vi "Clear.vi"(8 "error in (no error)":errorcluster, 11 "Image in":refnum<class "Image.lvclass">) -> (0 "error out":errorcluster, 3 "Image out":refnum<class "Image.lvclass">)   [LabVIEW 2020, in "RPI.SenseHat.Display.lvlib" / "Image.lvclass"]
doc: "Fills the image with black color."
uses:
  Image.lvclass
  Color/Color.lvclass
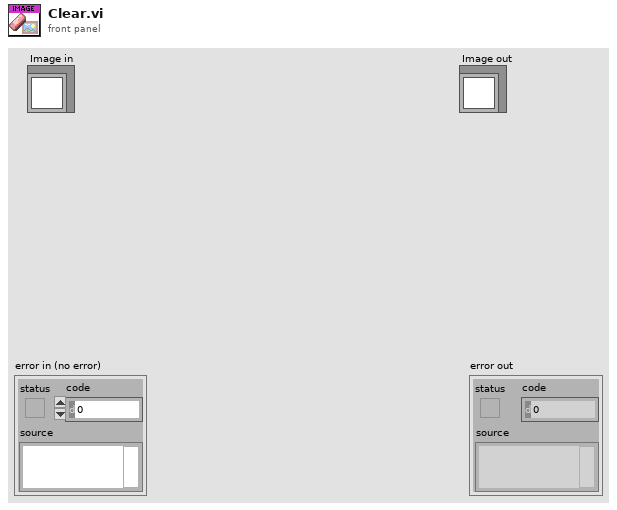
[diagram p1: front panel]
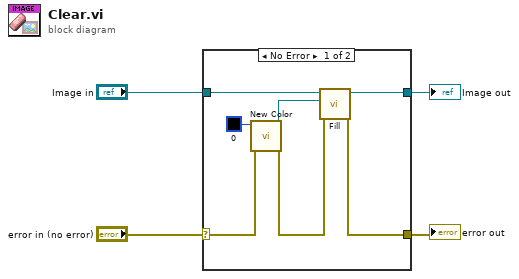
[diagram p0: block diagram]
diagram:
  n1 = case shown="No Error" "error in (no error)" {
    selector: "error in (no error)" -> [w7 w13]
    tunnel: [w9 w13] -> w3
    tunnel: [w10 w12] -> w1
    tunnel: "Image in" -> [w11 w12]
    frame No Error {
      n2 = call "New Color.vi"("error in (no error)"=w7, "Color Box"=u32 0) -> ("error out"=w6:errorcluster, "Color out"=w8:refnum<class "Color.lvclass">)  [unwired: 8 in]
      n3 = call "Fill.vi"("error in (no error)"=w6, "Color"=w8, "Image in"=w11) -> ("error out"=w9:errorcluster, "Image out"=w10:refnum<class "Image.lvclass">)  [unwired: 7 in]
    }
    frame Error {
    }
  }
  "error out" <- w3
  "Image out" <- w1
